vi "CreateChan-V3.vi"(8 "error in":errorcluster, 10 "Channel Info":T2=[{"Channel Name"="Untitled", "Sensitivity mV_EU"=1000.0, "EU"="V", "dB Ref EU"=1.0}, {"Channel Name"="Untitled", "Sensitivity mV_EU"=1000.0, "EU"="V", "dB Ref EU"=1.0}, {"Channel Name"="Untitled", "Sensitivity mV_EU"=1000.0, "EU"="V", "dB Ref EU"=1.0}, {"Channel Name"="Untitled", "Sensitivity mV_EU"=1000.0, "EU"="V", "dB Ref EU"=1.0}] {"dB Ref EU" format="%#.2p"; "Sensitivity mV_EU" format="%.2f"}, 11 "Dynamic FPGA Ref":T1) -> (0 "error out":errorcluster, 2 "Sampling Info":T3, 3 "Dynamic FPGA Ref Out":T1)   [LabVIEW 2015]
doc: "This VI collects and sends scaling coefficients as well as channel count to the FPGA. The number of elements in \"Channel Info\" must equal the number of channels acquired by the FPGA."
uses:
  <vilib>/NI/cRIO Wfm/SamplingInfo.ctl
  <vilib>/NI/cRIO Wfm/ChannelConfig.ctl
  <vilib>/NI/cRIO Wfm/DynamicFPGAref.ctl
  <vilib>/rvi/errors/niLvFpgaAdjustHostInterfaceError.vi
  <vilib>/Utility/error.llb/Error Cluster From Error Code.vi
  <vilib>/rvi/interface/nirviReadWriteControl/nirviReadWriteControl.xnode
  <vilib>/NI/cRIO Wfm/cRIO Wfm.lvlib
  <vilib>/rvi/interface/Simulation/niFpgaSimulationCallBeginRW.vi
  NiFpgaLv.dll
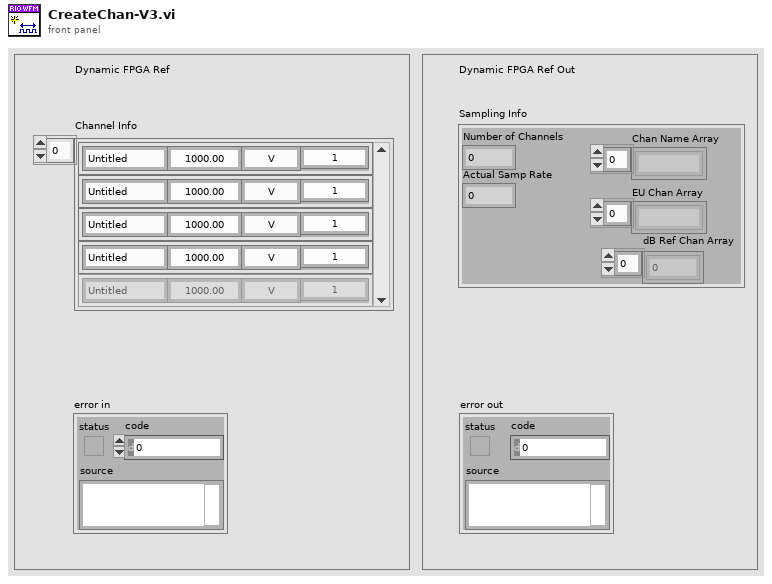
[diagram p1: front panel]
types:
  T1 = typedef "cRIO Wfm.lvlib/DynamicFPGAref.ctl" = refnum<k20>
  T2 = typedef "cRIO Wfm.lvlib/ChannelConfig.ctl" = cluster{"Channel Name":string, "Sensitivity mV_EU":dbl, "EU":string, "dB Ref EU":dbl}[]
  T3 = typedef "cRIO Wfm.lvlib/SamplingInfo.ctl" = cluster{"Number of Channels":i32, "Actual Samp Rate":dbl, "Chan Name Array":string[], "EU Chan Array":string[], "dB Ref Chan Array":dbl[]}
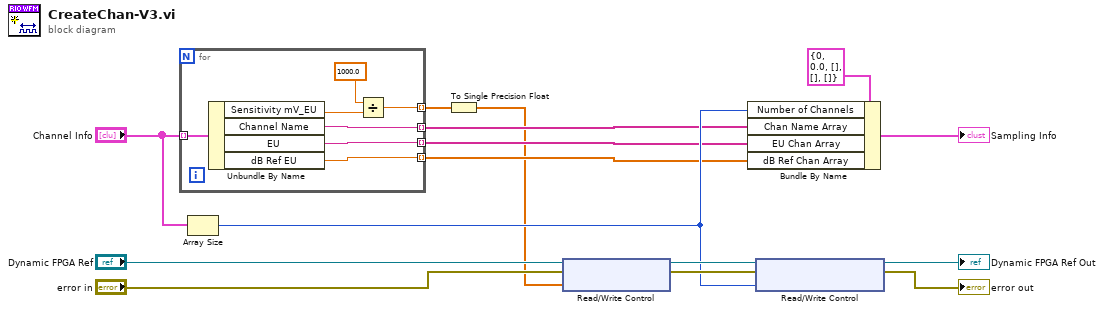
[diagram p0: block diagram]
diagram:
  n1 = for {
    tunnel: "Channel Info" -> [w21] mode=indexing
    tunnel: [w18] -> w6 mode=indexing
    tunnel: [w19] -> w7 mode=indexing
    tunnel: [w17] -> w5 mode=indexing
    tunnel: [w16] -> w2 mode=indexing
    n2 = Unbundle By Name(w21) -> ("Sensitivity mV_EU"=w20:dbl, "Channel Name"=w17:string, "EU"=w18:string, "dB Ref EU"=w19:dbl)
    n3 = Divide(x=1000.0 ("y"), y=w20) -> (x/y=w16:dbl)
  }
  n4 = Array Size(array="Channel Info") -> (size(s)=w9:i32)
  n5 = To Single Precision Float(number=w2) -> (single precision float=w1:sgl[])
  n6 = xnode "Read/Write Control"("FPGA VI Reference In"="Dynamic FPGA Ref", "error in"="error in", "Chan Scale Array"=w1) -> ("FPGA VI Reference Out"=w12:T1, "error out"=w11:errorcluster)
  n7 = Bundle By Name(cluster=T3 {"Number of Channels"=0, "Actual Samp Rate"=0.0, "Chan Name Array"=[], "EU Chan Array"=[], "dB Ref Chan Array"=[]} ("Sampling Info"), "Number of Channels"=w9, "Chan Name Array"=w5, "EU Chan Array"=w6, "dB Ref Chan Array"=w7) -> (→"Sampling Info":T3)
  n8 = xnode "Read/Write Control"("FPGA VI Reference In"=w12, "error in"=w11, "Number of Channels"=w9) -> ("FPGA VI Reference Out"=→"Dynamic FPGA Ref Out":T1, "error out"=→"error out":errorcluster)
